vi "Update-pane-by-index.vi"(8 "error in (no error)":errorcluster, 9 "Pane index":i32, 10 "Pane":T1, 11 "Panes in":T5) -> (0 "error out":errorcluster, 3 "Panes out":T5)   [LabVIEW 2013, in "SLMControl.lvlib" / "SC-UI.lvclass"]
uses:
  SC-UI.lvclass
  Panes-reference.ctl
  Pane-settings.ctl
  Pane-names.ctl
  Splitter-settings.ctl
  Splitter-names.ctl
  SC-UI.lvclass/SC-UI.ctl
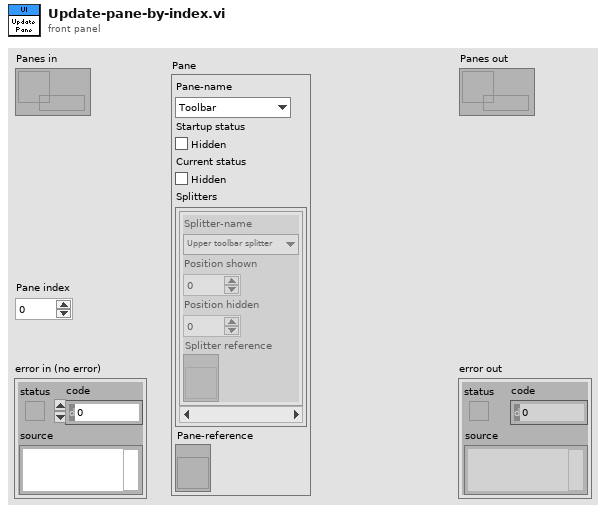
[diagram p1: front panel]
types:
  T1 = typedef "SLMControl.lvlib/SC-UI.lvclass/Pane-settings.ctl" = cluster{"Pane-name":T2, "Startup status":bool, "Current status":bool, "Splitters":T3[], "Pane-reference":refnum<vi>}
  T2 = typedef "SLMControl.lvlib/SC-UI.lvclass/Pane-names.ctl" = enum16{"Toolbar", "Help bar", "Toolbar lower border", "Center panel", "Main panel", "Status panel", "Status bar upper border", "General state bar", "Information bar"}
  T3 = typedef "SLMControl.lvlib/SC-UI.lvclass/Splitter-settings.ctl" = cluster{"Splitter-name":T4, "Position shown":i32, "Position hidden":i32, "Splitter reference":refnum<vi>}
  T4 = typedef "SLMControl.lvlib/SC-UI.lvclass/Splitter-names.ctl" = enum16{"Upper toolbar splitter", "Help bar splitter", "Lower toolbar splitter", "Upper status bar splitter", "Lower status bar splitter", "Left status bar splitter", "Status splitter"}
  T5 = typedef "SLMControl.lvlib/SC-UI.lvclass/Panes-reference.ctl" = refnum<data-value>
  T6 = typedef "SLMControl.lvlib/BC-UI.lvclass/Pane-settings.ctl" = cluster{"Pane-name":T7, "Startup status":bool, "Current status":bool, "Splitters":T8[], "Pane-reference":refnum<vi>}
  T7 = typedef "SLMControl.lvlib/BC-UI.lvclass/Pane-names.ctl" = enum16{"Toolbar", "Help bar", "Toolbar lower border", "Center panel", "Main panel", "Status panel", "Status bar upper border", "General state bar", "Information bar"}
  T8 = typedef "SLMControl.lvlib/BC-UI.lvclass/Splitter-settings.ctl" = cluster{"Splitter-name":T9, "Position shown":i32, "Position hidden":i32, "Splitter reference":refnum<vi>}
  T9 = typedef "SLMControl.lvlib/BC-UI.lvclass/Splitter-names.ctl" = enum16{"Upper toolbar splitter", "Help bar splitter", "Lower toolbar splitter", "Upper status bar splitter", "Lower status bar splitter", "Left status bar splitter", "Status splitter"}
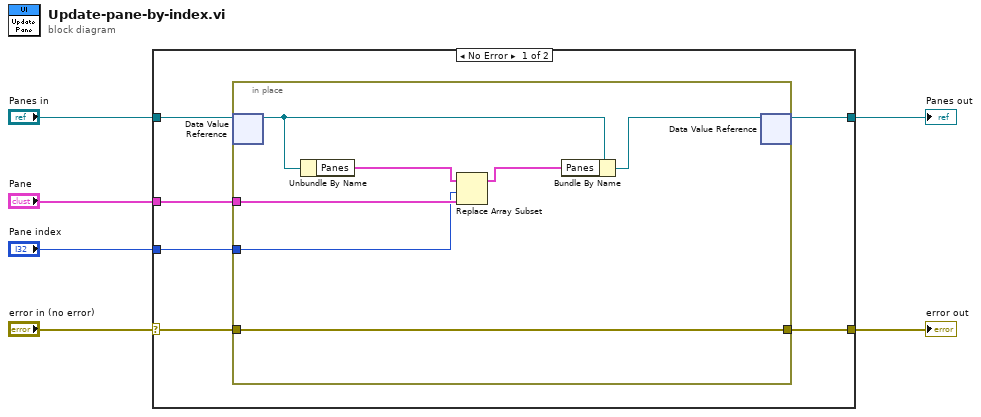
[diagram p0: block diagram]
diagram:
  n1 = case shown="No Error" "error in (no error)" {
    selector: "error in (no error)" -> [w8 w20]
    tunnel: [w7 w20] -> w5
    tunnel: [w9 w21] -> w3
    tunnel: "Panes in" -> [w12 w21]
    tunnel: "Pane index" -> [w10 _]
    tunnel: "Pane" -> [w11 _]
    frame No Error {
      n2 = in-place {
        in-place-border: w11 -> [w18]
        in-place-border: w10 -> [w17]
        in-place-border: w8 -> [w13]
        in-place-border: [w13] -> w7
        n3 = in-place-dvr #1(w12) -> (w15:refnum<class "SC-UI.lvclass">)  [unwired: 1 out]
        n4 = Unbundle By Name(w15) -> ("Panes"=w19:T6[])
        n5 = Replace Array Subset(array=w19, new element=w18, index=w17) -> (w16:T6[])
        n6 = Bundle By Name(cluster=w15, "Panes"=w16) -> (w14:refnum<class "SC-UI.lvclass">)
        n7 = in-place-dvr #1(w14) -> (w9:T5)  [unwired: 1 out]
      }
    }
    frame Error {
    }
  }
  "error out" <- w5
  "Panes out" <- w3
